vi "GetTxVoltage.vi"(6 "Legacy (f)?":bool, 8 "error in (no error)":errorcluster) -> (0 "error out":errorcluster, 2 "Detectors (V)":dbl[](array[numeric]))   [LabVIEW 2011]
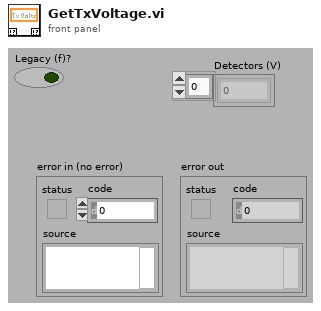
[diagram p1: front panel]
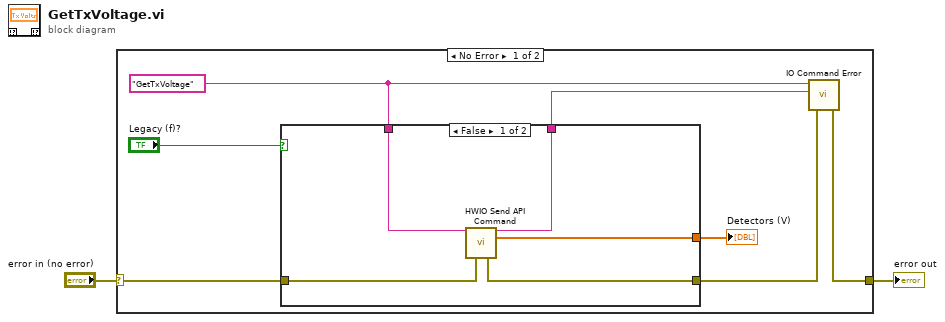
[diagram p0: block diagram]
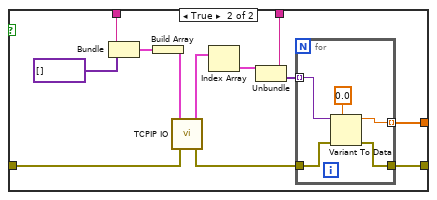
[diagram p2: hidden frame]
diagram:
  n1 = case shown="No Error" "error in (no error)" {
    selector: "error in (no error)" -> [w3 w32]
    tunnel: [w8 w32] -> w2
    frame No Error {
      w6 = "GetTxVoltage"
      n2 = case shown="False" "Legacy (f)?" {
        tunnel: w3 -> [w14 w24]
        tunnel: [w13 w22] -> w9
        tunnel: [w11 w21] -> w7
        tunnel: w6 -> [w10 w20]
        tunnel: [w12 w15] -> w5
        frame False {
          n3 = call "HWIO Send API Command.vi"("Action"=w10, "error in (no error)"=w14) -> ("Action out"=w11:string, "Double out"=w12:dbl[], "error out"=w13:errorcluster)  [unwired: 6 in, 5 out]
        }
        frame True {
          n4 = Bundle(w20, "appended array"=variant[] []) -> (w26:cluster{string, "appended array":variant[]})  [unwired: 1 out]
          n5 = Build Array(w26) -> (w17:cluster{string, "appended array":variant[]}[])
          n6 = call "TCPIP IO.vi"("error in (no error)"=w24, "Commands"=w17) -> ("error out"=w23:errorcluster, "Responses"=w19:cluster{string, variant[]}[])  [unwired: 1 in, 3 out]
          n7 = Index Array(array=w19) -> (element=w18:cluster{string, variant[]})  [unwired: 1 in]
          n8 = Unbundle(w18) -> (w21:string, w25:variant[])
          n9 = for {
            tunnel: [w31] -> w22
            tunnel: w23 -> [w30]
            tunnel: w25 -> [w29] mode=indexing
            tunnel: [w28] -> w15 mode=indexing
            n10 = Variant To Data(error in=w30, type=0.0, Variant=w29) -> (data=w28:dbl, error out=w31:errorcluster)
          }
        }
      }
      "Detectors (V)" <- w5
      n11 = call "IO Command Error.vi"("error in (no error)"=w9, "Command Returned (\"\")"=w7, "Command Sent (\"\")"=w6) -> ("error out"=w8:errorcluster)  [unwired: 4 out]
    }
    frame Error {
    }
  }
  "error out" <- w2
